vi "API Send Commands.vi"(4 "Timeout ms (30000)":i32=30000, 6 "Legacy (false)":bool, 7 "Commands":T4[](array[typedef]), 8 "error in (no error)":errorcluster, 9 "Token":string, 10 "API Port (80)":u16=80, 11 "API Server (localhost)":string="localhost") -> (0 "error out":errorcluster, 1 "Timed Out?":bool, 2 "Time To Response":u32, 5 "Responses":T1[](array[typedef]))   [LabVIEW 2011]
doc: "This VI is designed to send PIM API \"Commands\" and \"Token\" to the target PIM Web Engine (located at \"API Server\" and \"API Port\"). Set the \"Legacy\" boolean true to communicate with legacy PIM analyzers. The VI returns the \"Responses\" for each command."
uses:
  Controls/PIM.API.Command.Unique.ctl
  Controls/PIM.API.Response.Unique.ctl
  Controls/PIM.API.Response.Samples.ctl
  iQA Sweep Behavior.ctl
  Controls/PIM.API.REQUEST.ctl
  Controls/PIM.API.Command.Collection.ctl
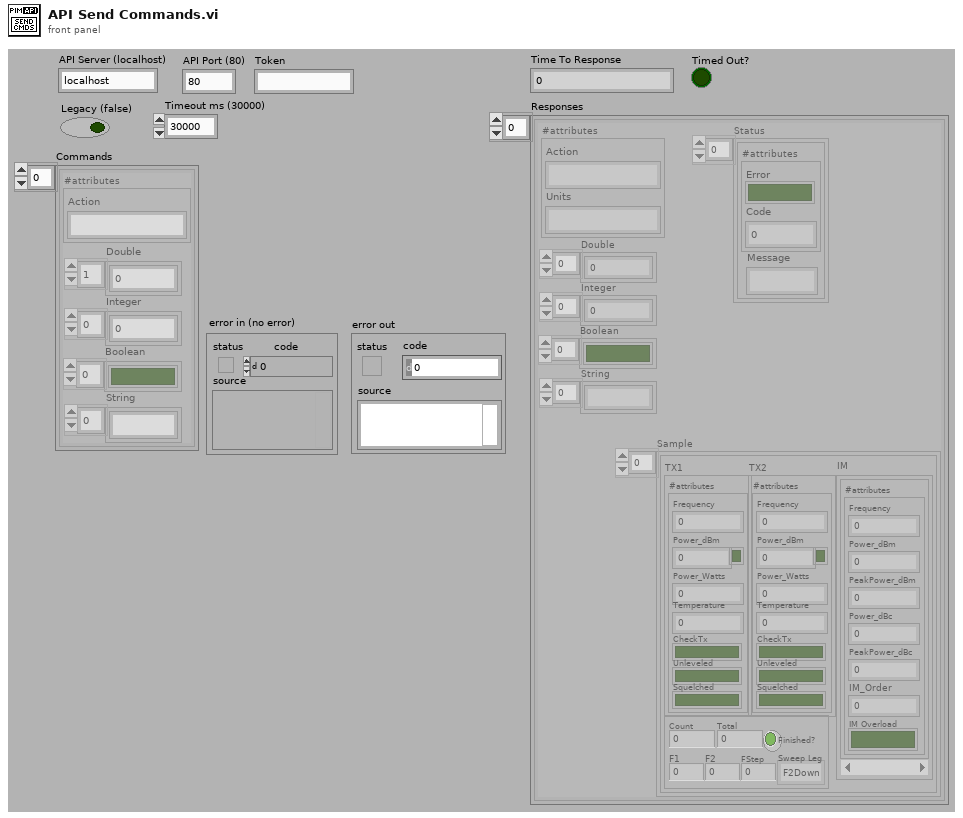
[diagram p1: front panel]
types:
  T1 = typedef "PIM.API.Response.Unique.ctl" = cluster{"#attributes":cluster{"Action":string, "Units":string}, "Double":dbl[], "Integer":i32[], "Boolean":bool[], "String":string[], "Sample":T2[], "Status":cluster{"#attributes":cluster{"Error":bool, "Code":i32}, "Message":string}[]}
  T2 = typedef "PIM.API.Response.Samples.ctl" = cluster{"TX1":cluster{"#attributes":cluster{"Frequency":dbl, "Power_dBm":dbl, "Power_Watts":dbl, "CheckTx":bool, "Unleveled":bool, "Squelched":bool, "Temperature":dbl, "ToneOn":bool}}, "TX2":cluster{"#attributes":cluster{"Frequency":dbl, "Power_dBm":dbl, "Power_Watts":dbl, "CheckTx":bool, "Unleveled":bool, "Squelched":bool, "Temperature":dbl, "ToneOn":bool}}, "IM":cluster{"#attributes":cluster{"Frequency":dbl, "Power_dBm":dbl, "PeakPower_dBm":dbl, "Power_dBc":dbl, "PeakPower_dBc":dbl, "IM_Order":u8, "IM Overload":bool}}[], "#attributes":cluster{"Count":u32, "Total":u32, "Finished?":bool, "Sweep Leg":T3, "F1":dbl, "F2":dbl, "FStep":dbl}}
  T3 = typedef "iQA Sweep Behavior.ctl" = enum16{"F2Down", "F1Up", "RxMultiIM"}
  T4 = typedef "PIM.API.Command.Unique.ctl" = cluster{"#attributes":cluster{"Action":string}, "Double":dbl[], "Integer":i32[], "Boolean":bool[], "String":string[]}
  T5 = typedef "PIM.API.REQUEST.ctl" = cluster{"#attributes":cluster{"xmlns":string, "xmlns:xsi":string, "xsi:schemaLocation":string}, "Commands":T6}
  T6 = typedef "PIM.API.Command.Collection.ctl" = cluster{"#attributes":cluster{"Token":string, "Legacy":bool}, "Command":T4[]}
  T7 = typedef "PIM.API.RESPONSE.ctl" = cluster{"#attributes":cluster{"xmlns":string, "xmlns:xsi":string, "xsi:schemaLocation":string}, "Responses":T8}
  T8 = typedef "PIM.API.Response.Collection.ctl" = cluster{"#attributes":cluster{"Legacy":bool}, "Response":T1[]}
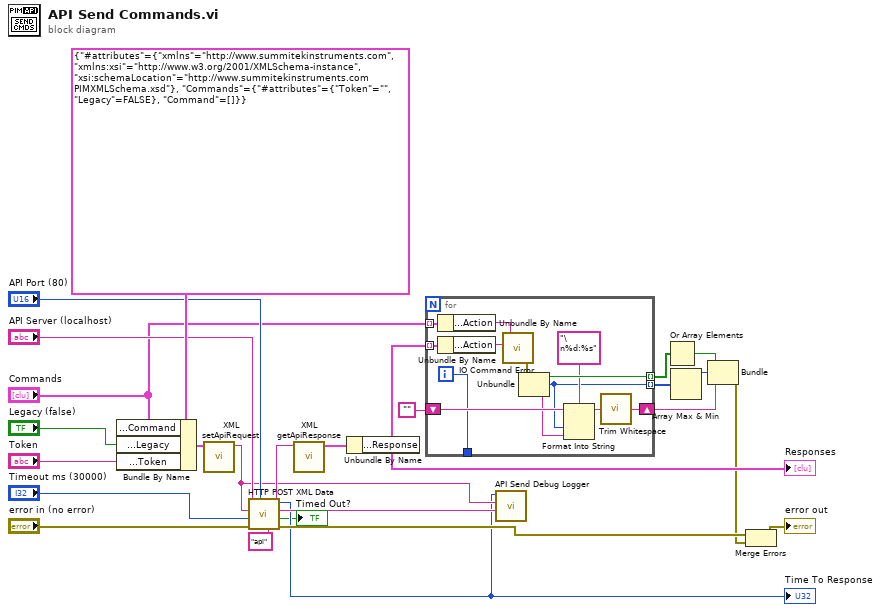
[diagram p0: block diagram]
diagram:
  n1 = Bundle By Name(cluster=T5 {"#attributes"={"xmlns"="http://www.summitekinstruments.com", "xmlns:xsi"="http://www.w3.org/2001/XMLSchema-instance", "xsi:schemaLocation"="http://www.summitekinstruments.com PIMXMLSchema.xsd"}, "Commands"={"#attributes"={"Token"="", "Legacy"=FALSE}, "Command"=[]}} ("PIM"), "Commands.Command"="Commands", "Commands.#attributes.Legacy"="Legacy (false)", "Commands.#attributes.Token"="Token") -> (w17:T5)
  n2 = call "XML setApiRequest.vi"("PIM API Request"=w17) -> ("Formatted XML"=w18:string)  [unwired: 9 in, 1 out]
  n3 = call "HTTP POST XML Data.vi"("webService/path (api)"="api", "port (80)"="API Port (80)", "error in (no error)"="error in (no error)", "Timeout ms (30000)"="Timeout ms (30000)", "XML Content"=w18, "address (localhost)"="API Server (localhost)") -> ("error out"=w11:errorcluster, "Timeout?"=→"Timed Out?":bool, "XML Response"=w19:string, "Comm Loop Time"=w2:u32)  [unwired: 2 in]
  "Time To Response" <- w2
  n4 = call "XML getApiResponse.vi"("Formatted XML"=w19) -> ("PIM API Response"=w15:T7)  [unwired: 10 in]
  n5 = Unbundle By Name(w15) -> ("Responses.Response"=w12:T1[])
  "Responses" <- w12
  n6 = for {
    tunnel: "Commands" -> [w38] mode=indexing
    tunnel: w12 -> [w37] mode=indexing
    shift-right: [w29] -> w4
    shift-left: "" -> [w30]
    tunnel: [w33] -> w8 mode=indexing
    tunnel: [w27] -> w6 mode=indexing
    tunnel: [w26] -> _
    i -> [w26]
    n7 = Unbundle By Name(w38) -> ("#attributes.Action"=w35:string)
    n8 = Unbundle By Name(w37) -> ("#attributes.Action"=w36:string)
    n9 = call "IO Command Error.vi"("Command Returned (\"\")"=w36, "Command Sent (\"\")"=w35) -> ("error out"=w34:errorcluster)  [unwired: 1 in, 4 out]
    n10 = Unbundle(w34) -> ("status"=w33:bool, "code"=w27:i32, "source"=w28:string)
    n11 = Format Into String(format string="\n%d:%s", initial string=w30, w27, w28) -> (resulting string=w32:string)  [unwired: 1 in, 1 out]
    n12 = call <vilib>:"Trim Whitespace.vi"("string"=w32) -> ("trimmed string"=w29:string)  [unwired: 1 in]
  }
  n13 = call "API Send Debug Logger.vi"("Response"=w19, "Command"=w18, "TimeToResponse"=w2) -> ()  [unwired: 8 in, 1 out]
  n14 = Or Array Elements(Boolean array=w8) -> (logical OR=w7:bool)
  n15 = Array Max & Min(array=w6) -> (max value=w5:i32)  [unwired: 3 out]
  n16 = Bundle(w7, w5, w4) -> (w3:errorcluster)  [unwired: 1 in]
  n17 = Merge Errors(w11, w3) -> (→"error out":errorcluster)
